vi "Global Connection Engine.vi"(6 "Connection Action":T1=enum."Get Connections", 7 "Signal Channel":variant, 9 "Signal Index":i32, 10 "QObject Refnum":u64) -> (2 "Signal Channels":variant[](array[variant]))   [LabVIEW 2013, in "Template.lvlib" / "LQWidgetEngine.lvclass"]
uses:
  LQWidgetEngine.lvclass
  Private/Connection Action.ctl
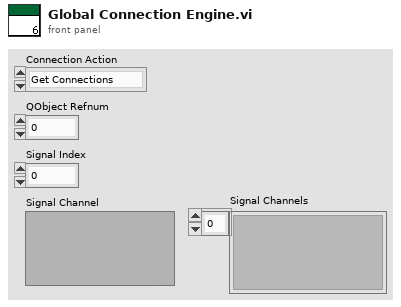
[diagram p1: front panel]
types:
  T1 = typedef "Template.lvlib/LQWidgetEngine.lvclass/Connection Action.ctl" = enum16{"Init", "Add Connection", "Get Connections", "Clean Up"}
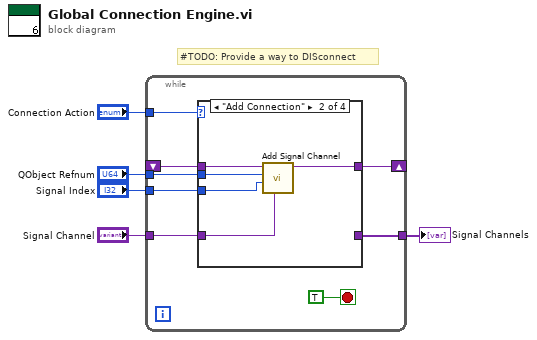
[diagram p0: block diagram]
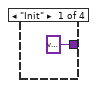
[diagram p2: hidden frame]
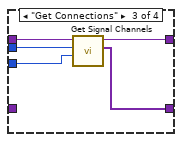
[diagram p3: hidden frame]
diagram:
  # "#TODO: Provide a way to DISconnect"
  n1 = while {
    tunnel: "Connection Action" -> [w13]
    shift-right: [w11] -> _
    shift-left: _ -> [w10]
    tunnel: "QObject Refnum" -> [w9]
    tunnel: "Signal Index" -> [w8]
    tunnel: "Signal Channel" -> [w7]
    tunnel: [w6] -> w1
    stop <- TRUE stop-if-true
    n2 = case shown="\"Add Connection\"" w13 {
      tunnel: [variant ("Dup. Signal Map") w19 w23 w25] -> w11
      tunnel: w10 -> [_ w18 w24 w25]
      tunnel: w9 -> [_ w17 w22 _]
      tunnel: w8 -> [_ w16 w21 _]
      tunnel: w7 -> [_ w15 _ _]
      tunnel: [_ _ w20 _] -> w6
      frame "Init" {
      }
      frame "Add Connection" {
        n3 = call "Add Signal Channel.vi"("Signal Channel"=w15, "Signal Index"=w16, "QObject Refnum"=w17, "Signal Map"=w18) -> ("Modified Signal Map"=w19:variant)  [unwired: 7 in]
      }
      frame "Get Connections" {
        n4 = call "Get Signal Channels.vi"("Signal Index"=w21, "QObject Refnum"=w22, "Signal Map"=w24) -> ("Signal Channels"=w20:variant[], "Dup. Signal Map"=w23:variant)  [unwired: 7 in]
      }
      frame "Clean Up" {
        # "#TODO: Clean up"
      }
    }
  }
  "Signal Channels" <- w1
